vi "컴퓨터Processㅑㅇ.vi"() -> ()   [LabVIEW 2014]
uses:
  Windows/System32/kernel32.dll
panel:
  out "반환 타입":i32
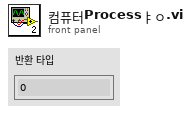
[diagram p1: front panel]
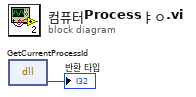
[diagram p0: block diagram]
diagram:
  n1 = dll-call lib="C:/Windows/System32/kernel32.dll" fn="GetCurrentProcessId"() -> ("반환 타입"=→"반환 타입":i32)  [unwired: 3 in, 2 out]
